vi "symulator_przyrzadu.vi"() -> ()   [LabVIEW 2021]
uses:
  stany_osc.ctl
  <vilib>/Analysis/NI_AALBase.lvlib
panel:
  in  "Przebieg":enum16{"sinus", "prostokąt", "trójkąt", "piła"}(ring)
  in  "Zapis wyników":bool
  in  "stop":bool
  out "Widmo częstotliwościowe":dbl[](graph)
  in  "Zerowanie fazy":bool
  in  "Amplituda zakłócenia":dbl(knob) scale=0.0..5.0
  in  "Współczynnik wypełnienia":dbl(knob) scale=25.0..75.0
  in  "Faza początkowa":dbl(knob) scale=0.0..90.0
  in  "Częstotliwość":dbl(knob)=1.0 scale=1.0..100.0
  in  "Amplituda":dbl(knob)=1.0 scale=1.0..10.0
  out "Przebieg czasowy":dbl[](graph)
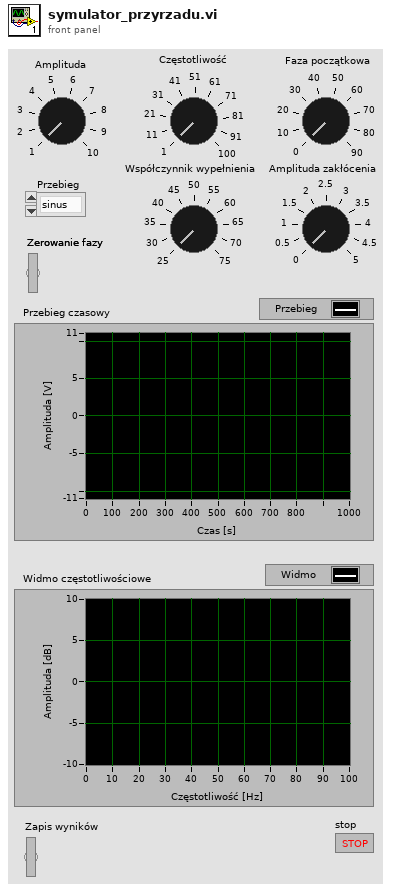
[diagram p1: front panel]
types:
  T1 = typedef "stany_osc.ctl" = enum16{"Init", "Idle", "Process", "Exit"}
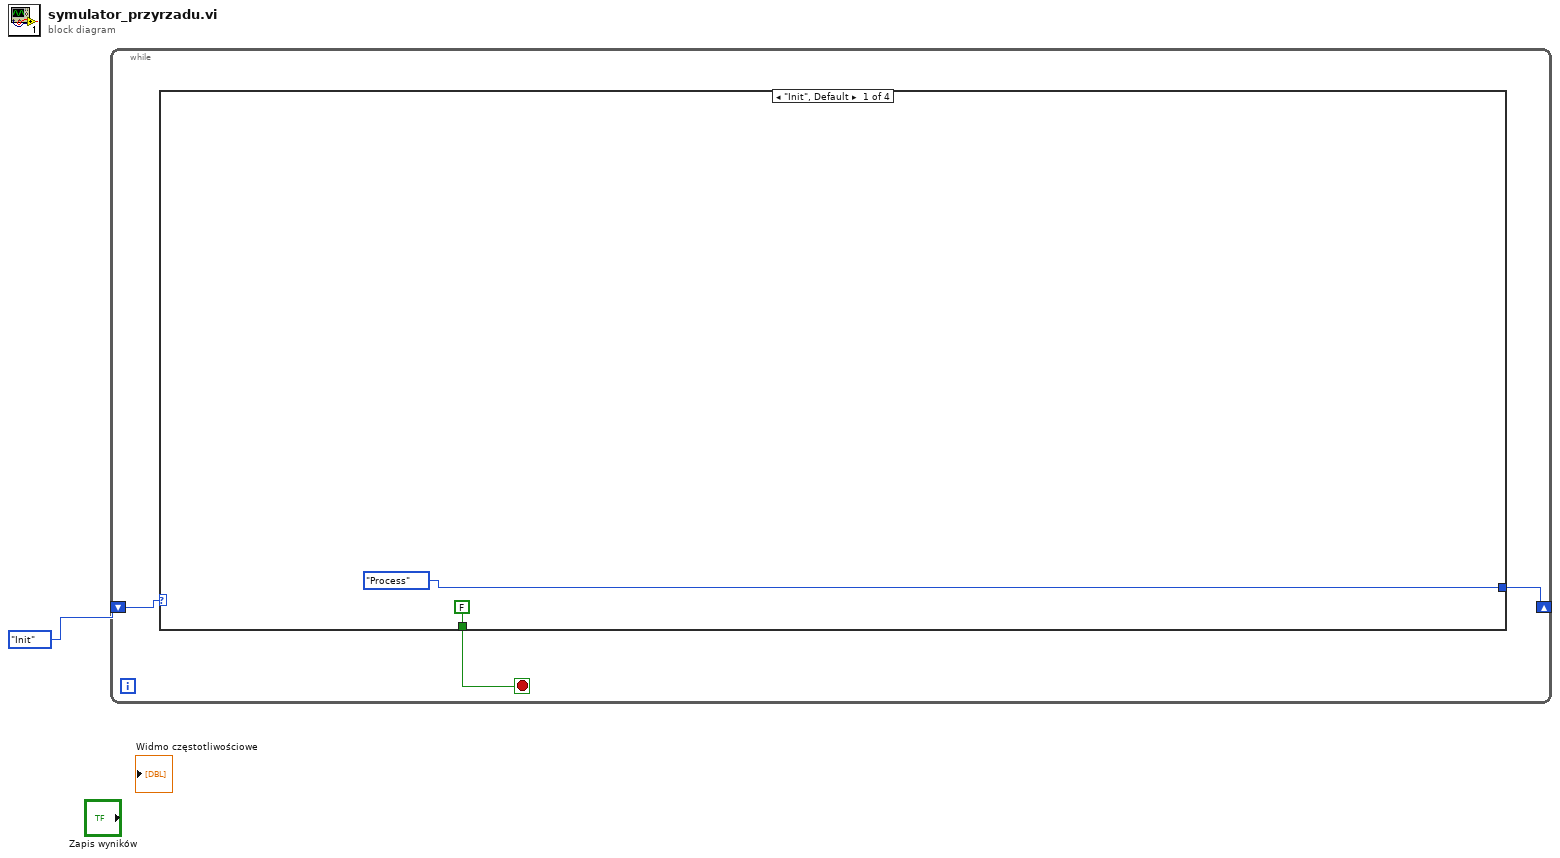
[diagram p0: block diagram]
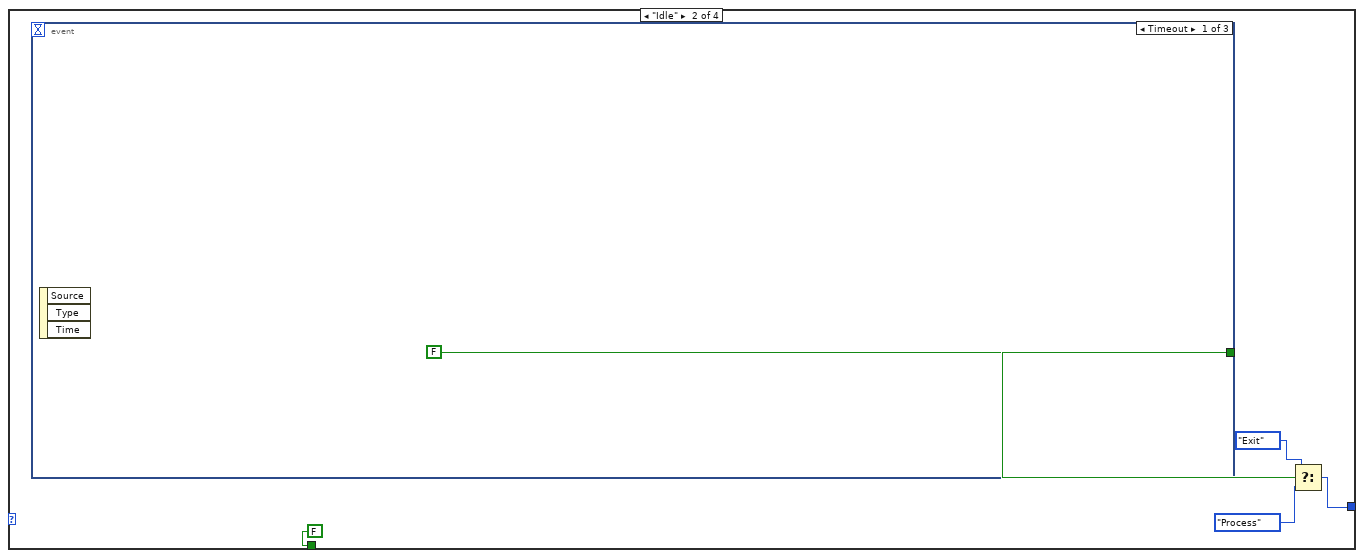
[diagram p2: hidden frame]
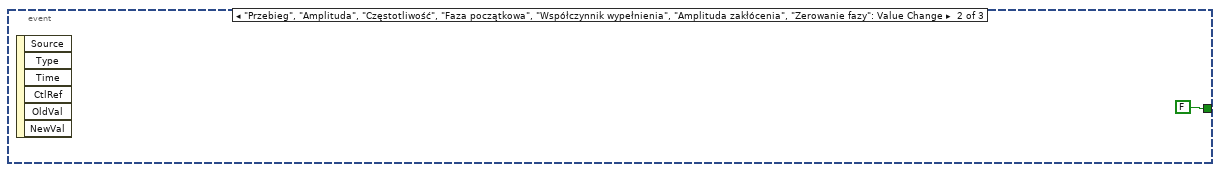
[diagram p3: hidden frame]
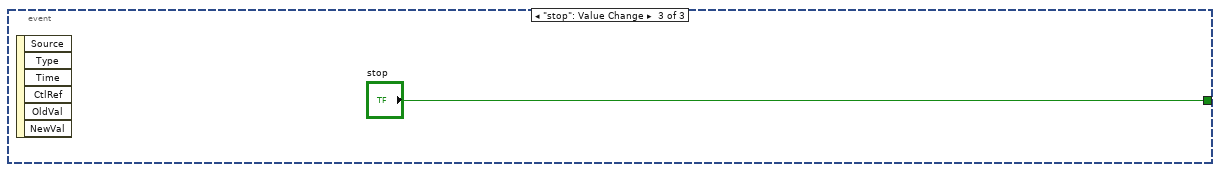
[diagram p4: hidden frame]
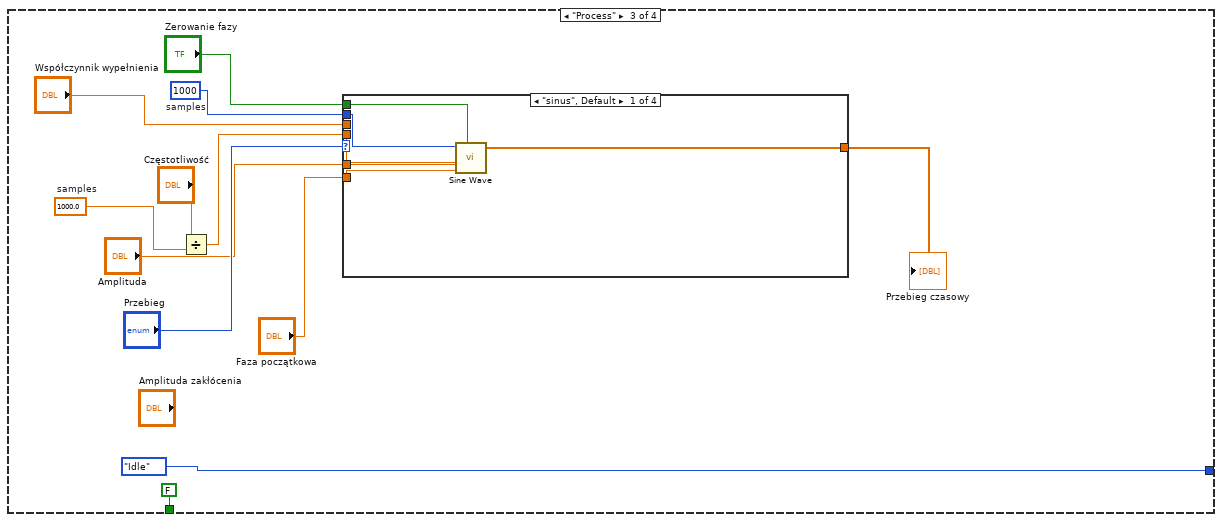
[diagram p5: hidden frame]
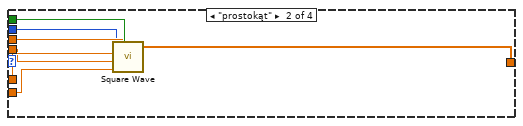
[diagram p6: hidden frame]
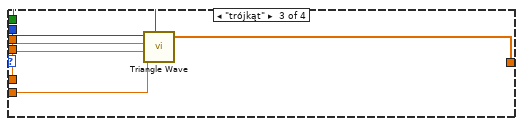
[diagram p7: hidden frame]
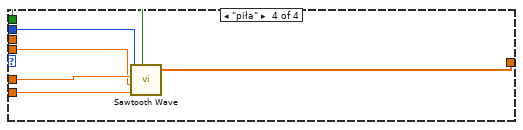
[diagram p8: hidden frame]
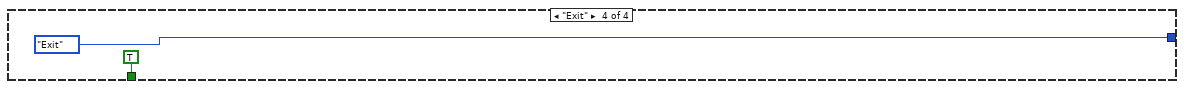
[diagram p9: hidden frame]
diagram:
  n1 = while {
    shift-right: [w3] -> _
    shift-left: stany_osc."Init" -> [w4]
    stop <- w2 stop-if-true
    n2 = case shown="\"Init\", Default" w4 {
      tunnel: [stany_osc."Process" w9 stany_osc."Idle" stany_osc."Exit"] -> w3
      tunnel: [FALSE FALSE FALSE TRUE] -> w2
      frame "Init", Default {
      }
      frame "Idle" {
        n3 = event shown="[0] Timeout" {
          selector: _ -> [_ _ _]
          dyn-events: _ -> [_ _ _]
          timeout: _ -> [_ _ _]
          tunnel: [FALSE ("stop") FALSE ("stop") "stop"] -> w7
          event Timeout {
            n4 = event-data() -> ()  [unwired: 1 in, 3 out]
          }
          event "Przebieg", "Amplituda", "Częstotliwość", "Faza początkowa", "Współczynnik wypełnienia", "Amplituda zakłócenia", "Zerowanie fazy": Value Change {
            n5 = event-data() -> ()  [unwired: 1 in, 6 out]
          }
          event "stop": Value Change {
            n6 = event-data() -> ()  [unwired: 1 in, 6 out]
          }
        }
        n7 = Select(t=stany_osc."Exit", s=w7, f=stany_osc."Process") -> (s? t:f=w9:T1)
      }
      frame "Process" {
        w16 = 1000.0  # samples
        w15 = 1000  # samples
        n8 = Divide(x="Częstotliwość", y=w16) -> (x/y=w19:dbl)
        n9 = case shown="\"sinus\", Default" "Przebieg" {
          tunnel: [w32 w39 w45 w51] -> w23
          tunnel: "Amplituda" -> [w31 w38 w41 w50]
          tunnel: "Zerowanie fazy" -> [w30 w37 w44 w49]
          tunnel: w15 -> [w28 w33 w43 w48]
          tunnel: w19 -> [w29 w36 w42 w47]
          tunnel: "Faza początkowa" -> [w27 w34 w40 w46]
          tunnel: "Współczynnik wypełnienia" -> [_ w35 _ _]
          frame "sinus", Default {
            n10 = call <vilib>:"Sine Wave.vi"("samples"=w28, "amplitude"=w31, "frequency"=w29, "phase in"=w27, "reset phase"=w30) -> ("sine wave"=w32:dbl[])  [unwired: 2 out]
          }
          frame "prostokąt" {
            n11 = call <vilib>:"Square Wave.vi"("samples"=w33, "reset phase"=w37, "amplitude"=w38, "frequency"=w36, "duty cycle (%)"=w35, "phase in"=w34) -> ("square wave"=w39:dbl[])  [unwired: 2 out]
          }
          frame "trójkąt" {
            n12 = call <vilib>:"Triangle Wave.vi"("samples"=w43, "amplitude"=w41, "frequency"=w42, "phase in"=w40, "reset phase"=w44) -> ("triangle wave"=w45:dbl[])  [unwired: 2 out]
          }
          frame "piła" {
            n13 = call <vilib>:"Sawtooth Wave.vi"("samples"=w48, "amplitude"=w50, "frequency"=w47, "phase in"=w46, "reset phase"=w49) -> ("sawtooth wave"=w51:dbl[])  [unwired: 2 out]
          }
        }
        "Przebieg czasowy" <- w23
      }
      frame "Exit" {
      }
    }
  }
